vi "LINC COSMOS Append Item.vi"(5 "ignore":bool, 6 "ID?":bool, 7 "macro":T1, 8 "error in (no error)":errorcluster, 9 "packet fields":T2, 10 "packet index":i32, 11 "packets in":T3[](array[typedef])) -> (0 "error out":errorcluster, 2 "item index":i32, 3 "packets out":T3[](array[typedef]))   [LabVIEW 2018, in "STEPkgDriver_LINC.lvlib"]
uses:
  STEPkgDriver_LINC.lvlib
  LINC Format Prototype.ctl
  LINC Packet.ctl
  LINC Packet Fields.ctl
  LINC Macro.ctl
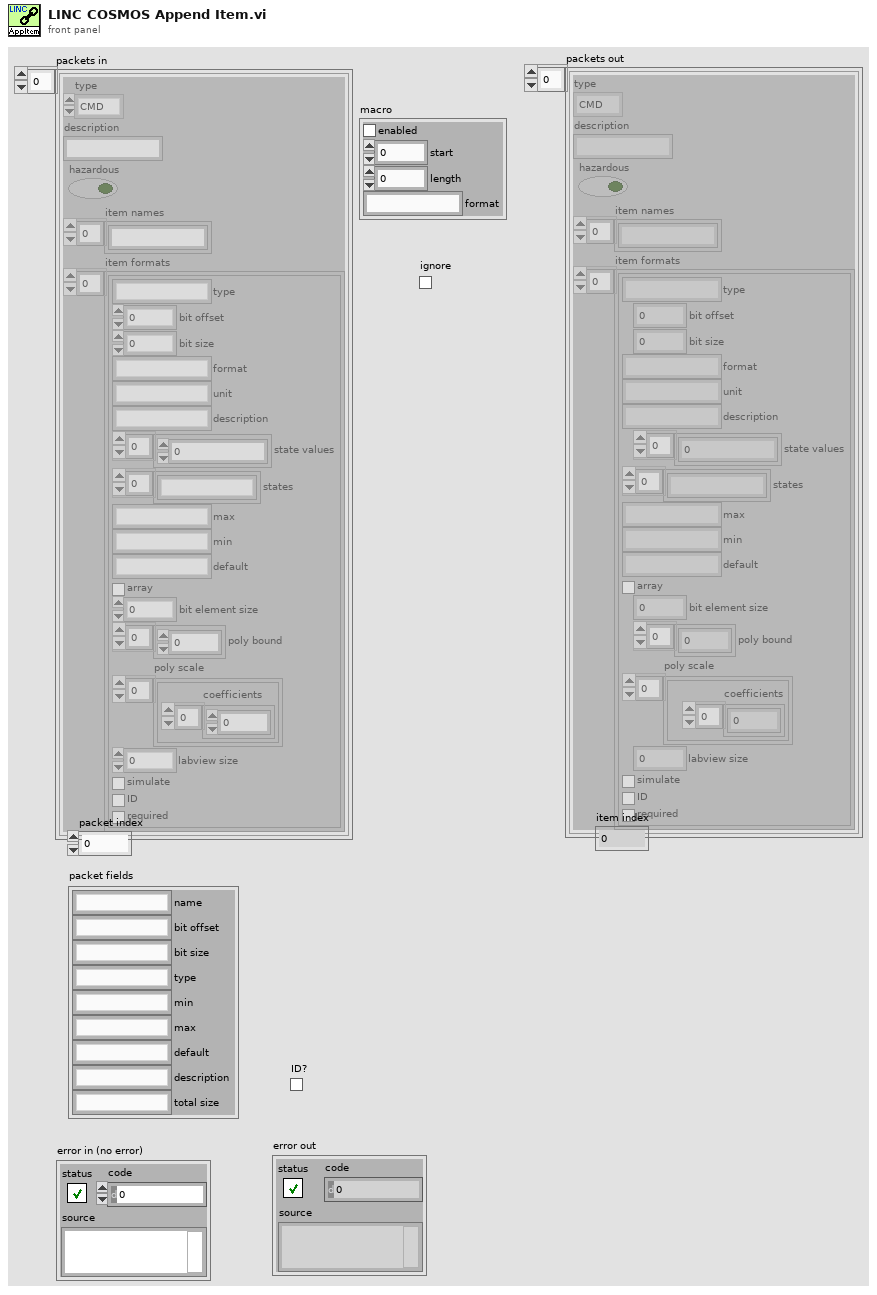
[diagram p1: front panel]
types:
  T1 = typedef "STEPkgDriver_LINC.lvlib/LINC Macro.ctl" = cluster{"enabled":bool, "start":i32, "length":i32, "format":string}
  T2 = typedef "STEPkgDriver_LINC.lvlib/LINC Packet Fields.ctl" = cluster{"name":string, "bit offset":string, "bit size":string, "type":string, "min":string, "max":string, "default":string, "description":string, "total size":string}
  T3 = typedef "STEPkgDriver_LINC.lvlib/LINC Packet.ctl" = cluster{"type":enum16{"CMD", "TLM"}, "description":string, "hazardous":bool, "item names":string[], "item formats":T4[]}
  T4 = typedef "STEPkgDriver_LINC.lvlib/LINC Format Prototype.ctl" = cluster{"type":string, "bit offset":i32, "bit size":i32, "format":string, "unit":string, "description":string, "state values":i64[], "states":string[], "max":string, "min":string, "default":string, "array":bool, "bit element size":i32, "poly bound":dbl[], "poly scale":cluster{"coefficients":dbl[]}[], "labview size":i32, "simulate":bool, "ID":bool, "required":bool}
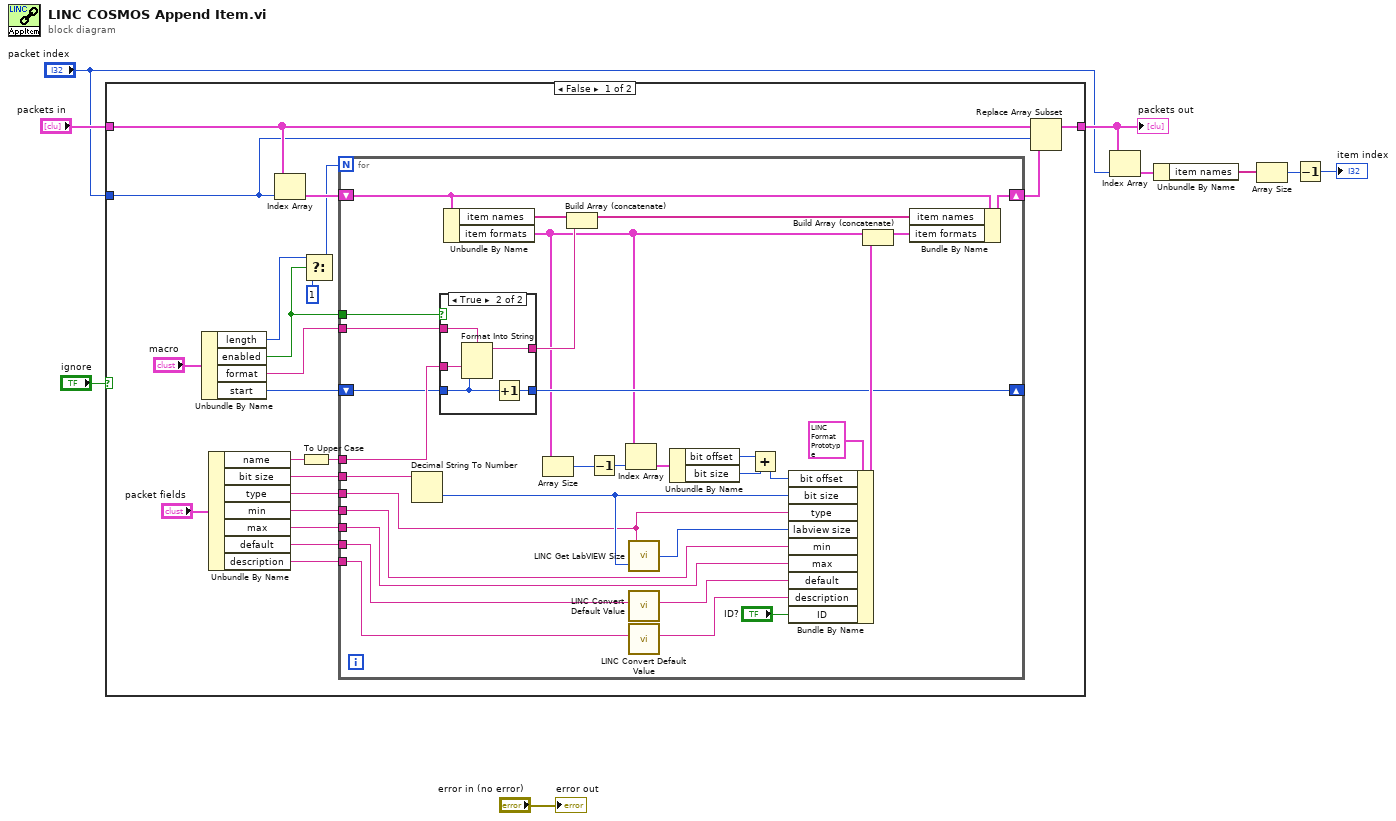
[diagram p0: block diagram]
diagram:
  n1 = case shown="False" "ignore" {
    tunnel: "packets in" -> [w29 w69]
    tunnel: [w28 w69] -> w3
    tunnel: "packet index" -> [w10 _]
    frame False {
      n2 = Unbundle By Name("macro") -> ("length"=w12:i32, "enabled"=w13:bool, "format"=w11:string, "start"=w16:i32)
      n3 = Unbundle By Name("packet fields") -> ("name"=w26:string, "bit size"=w25:string, "type"=w24:string, "min"=w23:string, "max"=w22:string, "default"=w21:string, "description"=w20:string)
      n4 = Index Array(array=w29, index=w10) -> (element=w18:T3)
      n5 = To Upper Case(1:w26) -> (0:w30:string)
      n6 = Select(t=w12, s=w13, f=1) -> (s? t:f=w14:i32)
      n7 = for {
        N: w14 -> [_]
        tunnel: w30 -> [w48]
        tunnel: w25 -> [w52]
        tunnel: w24 -> [w51]
        tunnel: w23 -> [w34]
        tunnel: w22 -> [w33]
        tunnel: w21 -> [w32]
        tunnel: w20 -> [w31]
        shift-right: [w49] -> w17
        shift-left: w18 -> [w50]
        shift-right: [w46] -> _
        shift-left: w16 -> [w47]
        tunnel: w11 -> [w45]
        tunnel: w13 -> [w44]
        n8 = Decimal String To Number(string=w52) -> (number=w58:i32)  [unwired: 2 in, 1 out]
        n9 = case shown="True" w44 {
          tunnel: w48 -> [w63 w66]
          tunnel: [w63 w68] -> w43
          tunnel: w45 -> [_ w67]
          tunnel: w47 -> [w62 w65]
          tunnel: [w62 w64] -> w46
          frame False {
          }
          frame True {
            n10 = Format Into String(format string=w67, w66, w65) -> (resulting string=w68:string)  [unwired: 2 in, 1 out]
            n11 = Increment(x=w65) -> (x+1=w64:i32)
          }
        }
        n12 = Unbundle By Name(w50) -> ("item names"=w55:string[], "item formats"=w35:T4[])
        n13 = Array Size(array=w35) -> (size(s)=w42:i32)
        n14 = Build Array (concatenate)(w55, w43) -> (w54:string[])
        n15 = Decrement(x=w42) -> (x-1=w38:i32)
        n16 = Index Array(array=w35, index=w38) -> (element=w39:T4)
        n17 = call "LINC Get LabVIEW Size.vi"("bit size"=w58, "type"=w51) -> ("labview size"=w57:i32)
        n18 = call "LINC Convert Default Value.vi"("default in"=w32) -> ("default out"=w59:string)  [unwired: 10 in]
        n19 = call "LINC Convert Default Value.vi"("default in"=w31) -> ("default out"=w56:string)  [unwired: 10 in]
        n20 = Unbundle By Name(w39) -> ("bit offset"=w40:i32, "bit size"=w41:i32)
        n21 = Add(x=w40, y=w41) -> (x+y=w37:i32)
        n22 = Bundle By Name(cluster=T4 {"type"="", "bit offset"=0, "bit size"=0, "format"="", "unit"="", "description"="", "state values"=[], "states"=[], "max"="", "min"="", "default"="", "array"=FALSE, "bit element size"=0, "poly bound"=[], "poly scale"=[], "labview size"=0, "simulate"=FALSE, "ID"=FALSE, "required"=FALSE} ("data"), "bit offset"=w37, "bit size"=w58, "type"=w51, "labview size"=w57, "min"=w34, "max"=w33, "default"=w59, "description"=w56, "ID"="ID?") -> (w60:T4)
        n23 = Build Array (concatenate)(w35, w60) -> (w36:T4[])
        n24 = Bundle By Name(cluster=w50, "item names"=w54, "item formats"=w36) -> (w49:T3)
      }
      n25 = Replace Array Subset(array=w29, new element=w17, index=w10) -> (w28:T3[])
    }
    frame True {
    }
  }
  "packets out" <- w3
  n26 = Index Array(array=w3, index="packet index") -> (element=w7:T3)
  n27 = Unbundle By Name(w7) -> ("item names"=w6:string[])
  n28 = Array Size(array=w6) -> (size(s)=w5:i32)
  n29 = Decrement(x=w5) -> (x-1=→"item index":i32)
  "error out" <- "error in (no error)"
